vi "test.vi"(1 "X":dbl, 2 "N":i32) -> (0 "Array":dbl[](array[numeric]))   [LabVIEW 2015]
uses:
  builds/test_prj/My DLL/SharedLib.dll
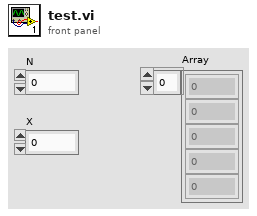
[diagram p1: front panel]
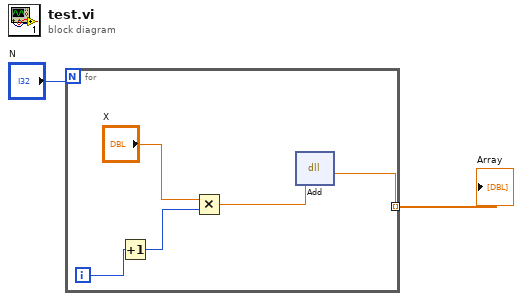
[diagram p0: block diagram]
diagram:
  n1 = for {
    N: "N" -> [_]
    tunnel: [w4] -> w1 mode=indexing
    i -> [w5]
    n2 = Increment(x=w5) -> ()  [unwired: 1 out]
    n3 = Multiply(x="X", y=w5) -> (x*y=w3:dbl)
    n4 = dll-call lib="D:/git/labview-demo/builds/test_prj/My DLL/SharedLib.dll" fn="Add"("X"=w3) -> ("X+Y"=w4:dbl)  [unwired: 4 in, 2 out]
  }
  "Array" <- w1
